vi "HP 3325A Function Gen.vi"(0 "marker":ext=5000000.0 format="%.3f", 1 "stop":ext=10000000.0 format="%.3f", 2 "start":ext=1000000.0 format="%.3f", 3 "sweep function (none:0)":u16(ring) items=["no sweep", "linear single", "linear cont.", "log single", "log cont."], 4 "sweep time (S)":ext=1.0 format="%.2f", 5 "modulation (off:0)":u16(ring) items=["off", "phase", "amplitude", "amp & phase"], 6 "frequency (Hz)":ext=1000.0 format="%.3f", 7 "offset (V)":ext format="%.2f", 8 "amplitude (V)":ext=1.0 format="%.4f", 9 "signal type (dc:0)":u16(ring) items=["dc ", "sine", "square", "triangle", "pos. ramp", "neg. ramp"]) -> ()   [LabVIEW 2014]
doc: "HP 3325A FUNCTION GENERATOR\n\nDEFAULT VALUES: Signal Type / DC Amplitude / 1 Volt Offset / 0 volts\n Frequency / 1KHz Sweep Time / 1 Second Modulation / Off \n Sweep function / No Sweep Sweep Frequency (Start) / 1MHz\n Sweep Frequency (Stop) / 10MHz Marker / 5MHz GPIB address / 1\n\nINTERACTIVE USE: The signal amplitude is entered in volts (peak to peak mode selected) with a range of .001 to 10 volts. The 'OFFSET' input ranges from -5 to 5 volts and should follow the limitations set out on pages 3-6 & 3-7 of the operating manual. Frequency can range from 1µHz to 60MHz with up to 11 significant digits. Frequencies above 21MHz will be outputted from the rear panel connector only. The sine function is the only function operative above 11MHz. The signal can be amplitude or phase modulated with a signal inputted from the rear panel. Additionally, the signal can also be frequency swept using the linear or log frequency sweep modes. The frequency sweep time can range from .01 to 99.99 seconds/sweep. The sweep can range from 1E-6 to < 21E6 Hz, log start frequency must be less than the stop frequency. A marker output is provided on the rear panel. This output is TTL and is approximately 400µS wide; the marker frequency should be at least 400µS before the stop frequency. With the 'SWEEP FUNCTION' switch set to 'No Sweep' the 'START', 'STOP', and 'MARKER' values have no effect on the signal. When the 'SWEEP FUNCTION' is set to one of the sweep functions, the 'FREQUENCY' input has no effect on the output. The output signal can be modulated and swept at the same time. Sweep errors are possible if the sweep frequency is to large for the selected function, sweep bandwidth is to small (log), sweep time is to short for chosen bandwidth, or the start frequency is greater than the stop frequency (log). The GPIB address is set to 1. This value can be changed by opening the diagram and changing the value in the string constant labeled 'GPIB Addr'.\n\nPROGRAMMATIC USE: All inputs to the 3325A instrument driver can be accessed from the connector pane. Slider switch input values are shown below. The example program included with this package shows the driver used programmatically. The ICON connector pane look like this:\n \n\n SIGNAL TYPE: 0 = DC\n 1 = SINE\n 2 = SQUARE\n 3 = TRIANGLE\n 4 = POSITIVE RAMP\n 5 = NEGATIVE RAMP\n\n MODULATION: 0 = MODULATION OFF\n 1 = PHASE\n 2 = AMPLITUDE\n 3 = AMPLITUDE & PHASE\n\n SWEEP FUNCTION: 0 = SWEEP OFF\n 1 = LINEAR SINGLE\n 2 = LINEAR CONTINUOUS\n 3 = LOG SINGLE\n 4 = LOG CONTINUOUS \n\nOPTIONS NOT INCLUDED: The High Voltage function was not available on our function generator and so was not added to this package. If your generator has this function it can be added to the command string before the amplitude is added. Additionally the Phase function was not added. Unused functions can be removed from the driver."
panel:
  # "HP 3325A function generator"
  # "sweep frequency (Hz)"
  # "© Copyright 1993 National Instruments Corporation.  ALL RIGHTS RESERVED."
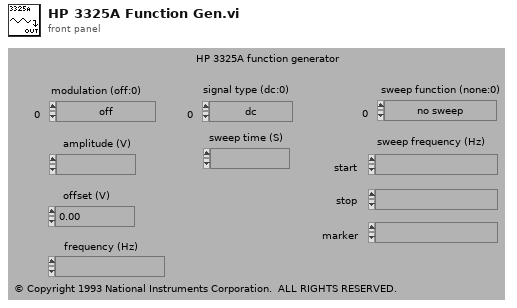
[diagram p1: front panel]
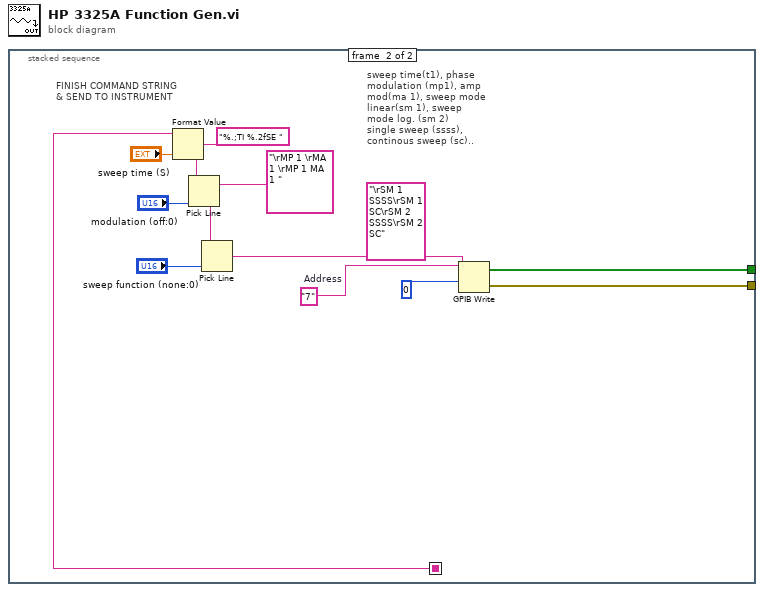
[diagram p0: block diagram]
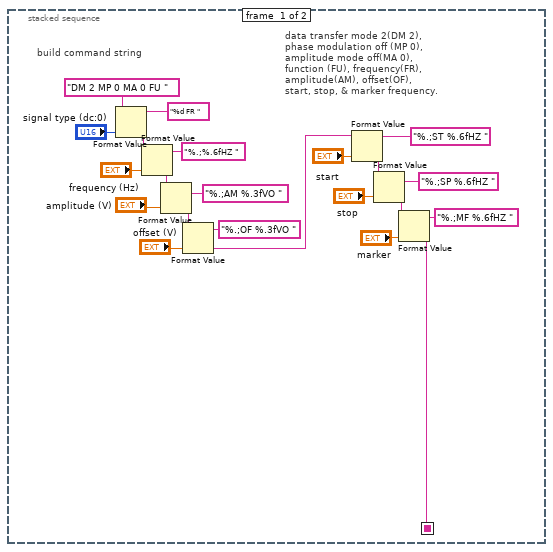
[diagram p2: hidden frame]
diagram:
  n1 = stacked-sequence {
    seq-local: [w22 _] -> [_ w31]
    tunnel: [_ w24] -> _
    tunnel: [_ w23] -> _
    frame #0 {
      # "data transfer mode 2(DM 2),\nphase modulation off (MP 0),\namplitude mode off(MA 0),\nfunction (FU), frequency(FR),\namplitude(AM), offset(OF),\nstart, stop, & marker frequency."
      # "build command string"
      n2 = Format Value(string ("")="DM 2 MP 0 MA 0 FU ", format string="%d FR ", value (0)="signal type (dc:0)") -> (output string=w2:string)
      n3 = Format Value(string ("")=w2, format string="%.;%.6fHZ ", value (0)="frequency (Hz)") -> (output string=w5:string)
      n4 = Format Value(string ("")=w5, format string="%.;AM %.3fVO ", value (0)="amplitude (V)") -> (output string=w7:string)
      n5 = Format Value(string ("")=w7, format string="%.;OF %.3fVO ", value (0)="offset (V)") -> (output string=w13:string)
      n6 = Format Value(string ("")=w13, format string="%.;ST %.6fHZ ", value (0)="start") -> (output string=w15:string)
      n7 = Format Value(string ("")=w15, format string="%.;SP %.6fHZ ", value (0)="stop") -> (output string=w19:string)
      n8 = Format Value(string ("")=w19, format string="%.;MF %.6fHZ ", value (0)="marker") -> (output string=w22:string)
    }
    frame #1 {
      w25 = "7"  # Address
      # "sweep time(t1), phase\nmodulation (mp1), amp\nmod(ma 1), sweep mode\nlinear(sm 1), sweep \nmode log. (sm 2)\nsingle sweep (ssss),\ncontinous sweep (sc).."
      # "FINISH COMMAND STRING\n& SEND TO INSTRUMENT"
      n9 = Format Value(string ("")=w31, format string="%.;TI %.2fSE ", value (0)="sweep time (S)") -> (output string=w33:string)
      n10 = Pick Line(string ("")=w33, multi-line string="\rMP 1 \rMA 1 \rMP 1 MA 1 ", line index="modulation (off:0)") -> (output string=w35:string)
      n11 = Pick Line(string ("")=w35, multi-line string="\rSM 1 SSSS\rSM 1 SC\rSM 2 SSSS\rSM 2 SC", line index="sweep function (none:0)") -> (output string=w30:string)
      n12 = GPIB Write(0:w25, 1:w30, 2:0) -> (5:w24:bool[], 6:w23:errorcluster)  [unwired: 1 in, 1 out]
    }
  }
